vi "rad_Get Target Info (Subnet) Wrapper.vi"(6 "reduce discovery timeout (T)":bool=TRUE, 8 "error in (no error)":errorcluster, 10 "only installable systems (T)":bool=TRUE) -> (0 "error out":errorcluster, 3 "target information":T1[](array[typedef]) {"Primary NIC"."IP Address Request Mode" items=["Static"=1, "DHCP/Link-Local"=2, "Link-Local Only"=4, "DHCP Only"=8]})   [LabVIEW 2016]
uses:
  TypeDefs/rad_Target Information.ctl
  TypeDefs/rad_Target Network Settings.ctl
  <vilib>/nisyscfg/Find Systems.vi
  <vilib>/nisyscfg/Close (System).vi
  <vilib>/nisyscfg/nisyscfg.lvlib
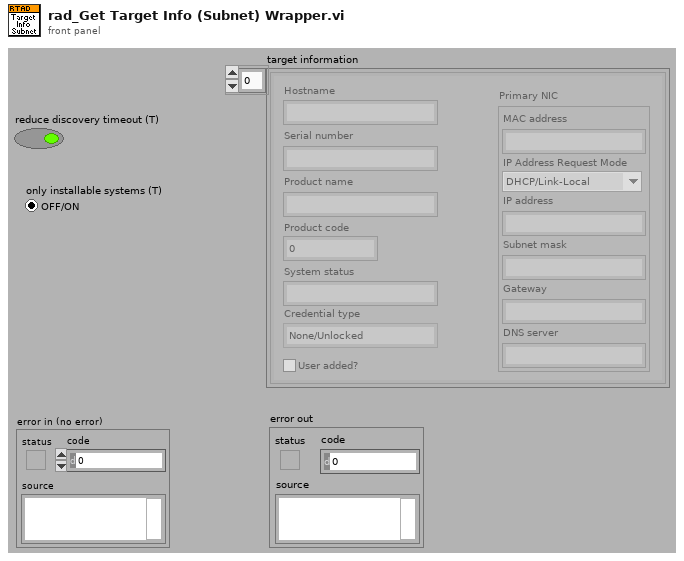
[diagram p1: front panel]
types:
  T1 = typedef "rad_Target Information.ctl" = cluster{"Hostname":string, "Serial number":string, "Product name":string, "Product code":i32, "System status":string, "Credential type":enum16{"None/Unlocked", "FTP Password", "NIAuth Credentials"}, "User added?":bool, "Primary NIC":T2}
  T2 = typedef "rad_Target Network Settings.ctl" = cluster{"MAC address":string, "IP Address Request Mode":i32, "IP address":string, "Subnet mask":string, "Gateway":string, "DNS server":string}
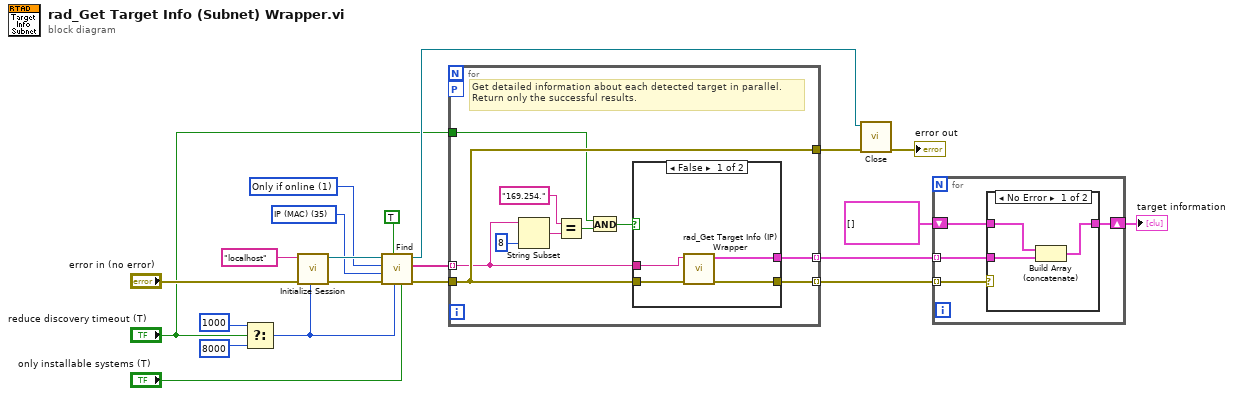
[diagram p0: block diagram]
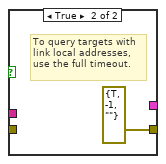
[diagram p3: hidden frame]
diagram:
  w17 = u32 35 items=["Hostname"=16, "Hostname (IP)"=18, "Hostname (MAC)"=19, "IP"=32, "IP (Hostname)"=33, "IP (MAC)"=35, "MAC"=48, "MAC (Hostname)"=49, "MAC (IP)"=50] ("output (hostname and IP)")
  w18 = u32 1 items=["None"=0, "Only if online"=1, "All"=3] ("include cached results (all)")
  n1 = Select(t=u32 1000, s="reduce discovery timeout (T)", f=u32 8000) -> (s? t:f=w1:u32)
  n2 = call <vilib>:"Initialize Session.vi"("Connect Timeout (4000 ms)"=w1, "error in (no error)"="error in (no error)", "Target (localhost)"="localhost") -> ("error out"=w16:errorcluster, "Session out"=w20:refnum<k21>)  [unwired: 7 in]
  n3 = call-poly <vilib>:"Find.vi"("Only Installable Systems (F)"="only installable systems (T)", "Timeout (4000 ms)"=w1, "Detect Online Systems (T)"=TRUE ("detect online systems (T)"), "error in (no error)"=w16, "Output (Hostname and IP)"=w17, "Include Cached Results (all)"=w18, "Session in (localhost)"=w20) -> ("error out"=w13:errorcluster, "Detected Systems"=w15:string[], "Session out"=w11:refnum<k21>)  [unwired: 2 in]
  n4 = for {
    tunnel: w15 -> [w28] mode=indexing
    tunnel: w13 -> [w31]
    tunnel: [w31] -> w12
    workers-P: _ -> [_]
    tunnel: [w30] -> w8 mode=indexing
    tunnel: [w29] -> w9 mode=indexing
    tunnel: "reduce discovery timeout (T)" -> [w22]
    # "Get detailed information about each detected target in parallel.\nReturn only the successful results."
    n5 = String Subset(string=w28, length (rest)=8 ("length (rest)")) -> (substring=w25:string)  [unwired: 1 in]
    n6 = Equal?(x="169.254.", y=w25) -> (x = y?=w23:bool)
    n7 = And(x=w22, y=w23) -> (x .and. y?=w24:bool)
    n8 = case shown="False" w24 {
      tunnel: w31 -> [w35 _]
      tunnel: [w34 errorcluster {"status"=TRUE, "code"=-1, "source"=""} ("error out")] -> w30
      tunnel: [w33 _] -> w29
      tunnel: w28 -> [w32 _]
      frame False {
        n9 = call "rad_Get Target Info (IP) Wrapper.vi"("error in (no error)"=w35, "target address"=w32) -> ("error out"=w34:errorcluster, "Target settings"=w33:T1)  [unwired: 8 in]
      }
      frame True {
        # "To query targets with\nlink local addresses,\nuse the full timeout."
      }
    }
  }
  n10 = call-poly <vilib>:"Close.vi"("error in (no error)"=w12, "Session in"=w11) -> ("error out"=→"error out":errorcluster)  [unwired: 9 in]
  n11 = for {
    tunnel: w9 -> [w38] mode=indexing
    tunnel: w8 -> [w40] mode=indexing
    shift-right: [w37] -> w6
    shift-left: T1[] [] -> [w39]
    n12 = case shown="No Error" w40 {
      tunnel: w39 -> [w43 w44]
      tunnel: w38 -> [w42 _]
      tunnel: [w41 w44] -> w37
      frame No Error {
        n13 = Build Array (concatenate)(w43, w42) -> (w41:T1[])
      }
      frame Error {
      }
    }
  }
  "target information" <- w6
